vi "string_inteira_carater.vi"(11 "String in":string) -> (3 "String out":string)   [LabVIEW 2019]
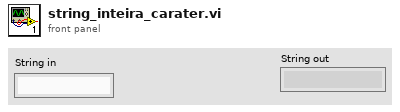
[diagram p1: front panel]
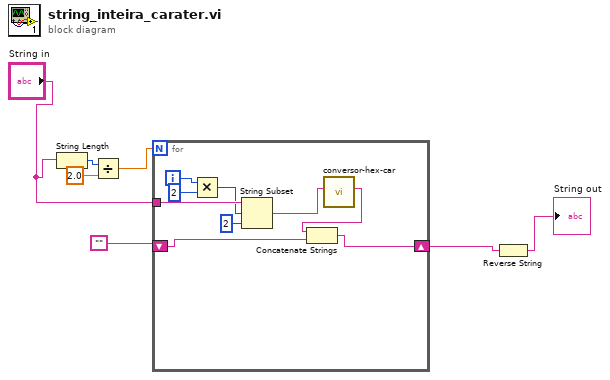
[diagram p0: block diagram]
diagram:
  n1 = String Length(string="String in") -> (length=w6:i32)
  n2 = Divide(x=w6, y=2.0) -> (x/y=w5:dbl)
  n3 = for {
    N: w5 -> [_]
    tunnel: "String in" -> [w16]
    shift-right: [w10] -> w3
    shift-left: "" -> [w11]
    i -> [w14]
    n4 = Multiply(x=w14, y=2) -> (x*y=w12:i32)
    n5 = String Subset(string=w16, offset (0)=w12, length (rest)=2 ("length (rest)")) -> (substring=w9:string)
    n6 = call "conversor-hex-car.vi"("String"=w9) -> ("String 2"=w8:string)  [unwired: 10 in]
    n7 = Concatenate Strings(w8, w11) -> (w10:string)
  }
  n8 = Reverse String(1:w3) -> (0:→"String out":string)
